vi "cRIO AI data1.vi"(0 "I":dbl, 1 "Input cluster":T1, 5 "error in (no error)":errorcluster, 6 "Chan 0":bool=TRUE, 7 "Scale factor0":dbl, 8 "Chan 1":bool, 9 "Scale factor1":dbl, 10 "Chan 2":bool, 11 "Scale factor2":dbl, 12 "Chan 3":bool, 13 "Scale factor3":dbl) -> (14 "Output data":dbl[](array[numeric]), 19 "error out":errorcluster)   [LabVIEW 2024]
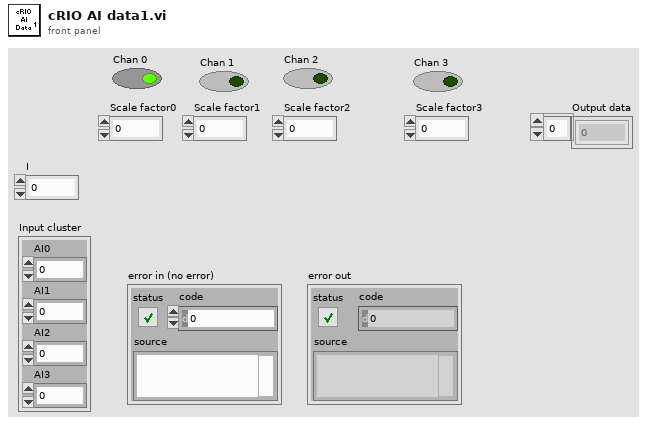
[diagram p1: front panel]
types:
  T1 = cluster{"AI0":dbl, "AI1":dbl, "AI2":dbl, "AI3":dbl}
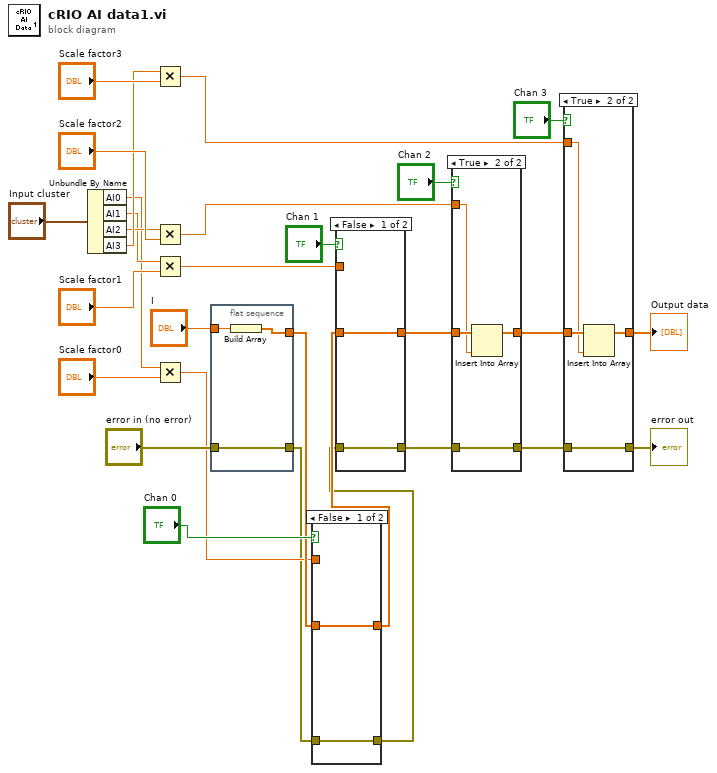
[diagram p0: block diagram]
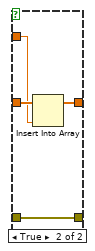
[diagram p2: hidden frame]
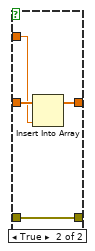
[diagram p5: hidden frame]
diagram:
  n1 = Unbundle By Name("Input cluster") -> ("AI0"=w8:dbl, "AI1"=w9:dbl, "AI2"=w10:dbl, "AI3"=w11:dbl)
  n2 = Multiply(x=w11, y="Scale factor3") -> (x*y=w23:dbl)
  n3 = Multiply(x=w10, y="Scale factor2") -> (x*y=w22:dbl)
  n4 = Multiply(x=w9, y="Scale factor1") -> (x*y=w21:dbl)
  n5 = Multiply(x=w8, y="Scale factor0") -> (x*y=w3:dbl)
  n6 = flat-sequence {
    tunnel: "error in (no error)" -> [w32]
    tunnel: [w32] -> w2
    tunnel: [w31] -> w5
    tunnel: "I" -> [w30]
    frame #0 {
      n7 = Build Array(w30) -> (w31:dbl[])
    }
  }
  n8 = case shown="False" "Chan 0" {
    tunnel: w2 -> [w33 w38]
    tunnel: [w33 w38] -> w1
    tunnel: w5 -> [w34 w37]
    tunnel: w3 -> [_ w36]
    tunnel: [w34 w35] -> w4
    frame False {
    }
    frame True {
      n9 = Insert Into Array(array=w37, new element=w36) -> (w35:dbl[])  [unwired: 1 in]
    }
  }
  n10 = case shown="False" "Chan 1" {
    tunnel: w1 -> [w39 w44]
    tunnel: [w39 w44] -> w16
    tunnel: w4 -> [w40 w43]
    tunnel: w21 -> [_ w42]
    tunnel: [w40 w41] -> w19
    frame False {
    }
    frame True {
      n11 = Insert Into Array(array=w43, new element=w42) -> (w41:dbl[])  [unwired: 1 in]
    }
  }
  n12 = case shown="True" "Chan 2" {
    tunnel: w16 -> [w45 w50]
    tunnel: [w45 w50] -> w17
    tunnel: w19 -> [w46 w49]
    tunnel: w22 -> [_ w48]
    tunnel: [w46 w47] -> w20
    frame False {
    }
    frame True {
      n13 = Insert Into Array(array=w49, new element=w48) -> (w47:dbl[])  [unwired: 1 in]
    }
  }
  n14 = case shown="True" "Chan 3" {
    tunnel: w17 -> [w51 w53]
    tunnel: w20 -> [w52 w56]
    tunnel: w23 -> [_ w55]
    tunnel: [w52 w54] -> w26
    tunnel: [w51 w53] -> w25
    frame False {
    }
    frame True {
      n15 = Insert Into Array(array=w56, new element=w55) -> (w54:dbl[])  [unwired: 1 in]
    }
  }
  "Output data" <- w26
  "error out" <- w25
